vi "Config_Input.vi"(8 "Start":bool, 10 "Throttle":dbl, 11 "Steering":dbl) -> (2 "Speed":dbl, 3 "Steer":dbl)   [LabVIEW 2012]
uses:
  <vilib>/Simulation/Implementation/Shared/SIMSCR Execution Mode.ctl
  <vilib>/Simulation/Scripting/Companion Diagram/SimConfigNode/SimParams.ctl
  <vilib>/Simulation/Scripting/Companion Diagram/SimConfigNode/_simSolvers.ctl
  <vilib>/Simulation/Param Hierarchy/Typedefs/SIMPH Param Control Actions.ctl
  <vilib>/Simulation/Implementation/Shared/NILVSim_ParamChanged.vi
  <vilib>/Simulation/SignalArithmetic/Implementation/NILVSim Gain.llb/SIM Gain (scalar).vi
  <vilib>/Simulation/Utility/Implementation/NILVSim Memory.llb/NILVSim Memory (core).vi
  <vilib>/Simulation/Nonlinear/Implementation/NILVSim RateLimiter.llb/SIM RateLimiter (scalar).vi
  <vilib>/Simulation/Nonlinear/Implementation/NILVSim Saturation.llb/SIM Saturation (scalar).vi
  <vilib>/Simulation/Implementation/Shared/NILVSim_Manager.vi
  <vilib>/Simulation/Implementation/Shared/NILVSim_FinalizeModel.vi
  <vilib>/Simulation/Implementation/Shared/SIM Unbundle Sim Info.vi
  <vilib>/Utility/error.llb/Clear Errors.vi
  <vilib>/Simulation/Implementation/Shared/NILVSim_GetModelError.vi
  <vilib>/Simulation/Implementation/Shared/SIM SimErrorHandler.vi
  <vilib>/Simulation/Implementation/Shared/SIM Bundle Sim Info.vi
  <vilib>/Simulation/Implementation/Shared/SIMSH Read Queue.vi
  <vilib>/Simulation/Implementation/Shared/NILVSim_Initialize.vi
  <vilib>/Simulation/Utility/Implementation/NILVSim Get Time and IsAcceptedStep.vi
  <vilib>/Simulation/Scripting/Companion Diagram/SimConfigNode/SimDog.xnode
  <vilib>/Simulation/Implementation/XNodeFramework/SimXNode/SimX.xnode
  <vilib>/Simulation/Implementation/Shared/NI_SIM_Implementation.lvlib
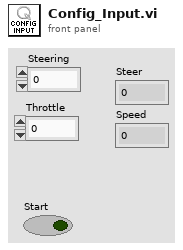
[diagram p1: front panel]
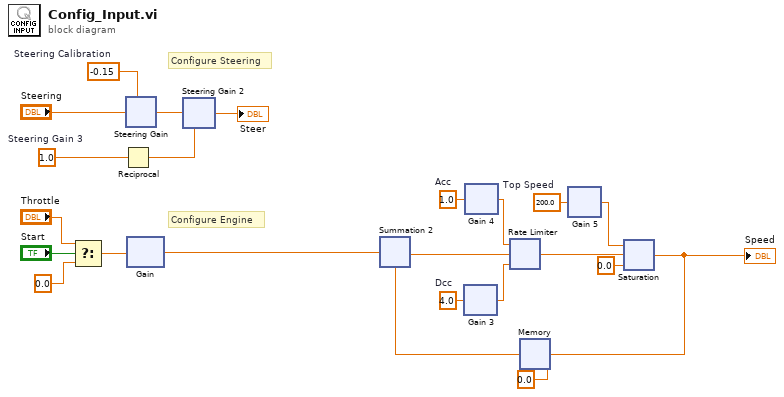
[diagram p0: block diagram]
diagram:
  w6 = 1.0  # Steering Gain 3
  w10 = 200.0  # Top Speed
  w12 = 1.0  # Acc
  w13 = 4.0  # Dcc
  w19 = -0.15  # Steering Calibration
  # "Configure Engine"
  # "Configure Steering"
  n1 = Select(t="Throttle", s="Start", f=0.0) -> (s? t:f=w18:dbl)
  n2 = Reciprocal(x=w6) -> (1/x=w5:dbl)
  n3 = xnode ("Steering Gain")("gain"=w19, "input"="Steering") -> ("output"=w8:dbl)  [unwired: 2 in]
  n4 = xnode ("Gain")("input"=w18) -> ("output"=w2:dbl)  [unwired: 3 in]
  n5 = xnode ("Steering Gain 2")("gain"=w5, "input"=w8) -> ("output"=→"Steer":dbl)  [unwired: 2 in]
  n6 = xnode ("Gain 3")("input"=w13) -> ("output"=w14:dbl)  [unwired: 3 in]
  n7 = xnode ("Gain 4")("input"=w12) -> ("output"=w11:dbl)  [unwired: 3 in]
  n8 = xnode ("Gain 5")("input"=w10) -> ("output"=w9:dbl)  [unwired: 3 in]
  n9 = xnode ("Summation 2")("Operand1"=w2, "Operand2"=w16) -> ("Result"=w3:dbl)
  n10 = xnode "Rate Limiter"("positive slew rate"=w11, "input"=w3, "negative slew rate"=w14) -> ("output"=w4:dbl)  [unwired: 2 in]
  n11 = xnode "Saturation"("upper limit"=w9, "input"=w4, "lower limit"=0.0) -> ("output"=w1:dbl)  [unwired: 2 in]
  "Speed" <- w1
  n12 = xnode "Memory"("input"=w1, "initial value"=0.0) -> ("output"=w16:dbl)  [unwired: 4 in]
